vi "state buffer.vi"(8 "change command":T2, 9 "write state":T1={"command"=enum."Idle", "start time (ms)"=0, "Channel Indices"=[], "Scans per Sample"=1} {"Scans per Sample" min=1}, 10 "connection":refnum<k5>, 11 "command":T3(ring)) -> (0 "state array":T1[](array[typedef]) {"Scans per Sample" min=1}, 1 "connections":refnum<k5>[](array[refnum]), 2 "clients":i32)   [LabVIEW 2012]
uses:
  command cluster.ctl
  command.ctl
panel:
  in  "add state":T1={"command"=enum."Idle", "start time (ms)"=0, "Channel Indices"=[], "Scans per Sample"=1} {"Scans per Sample" min=1}
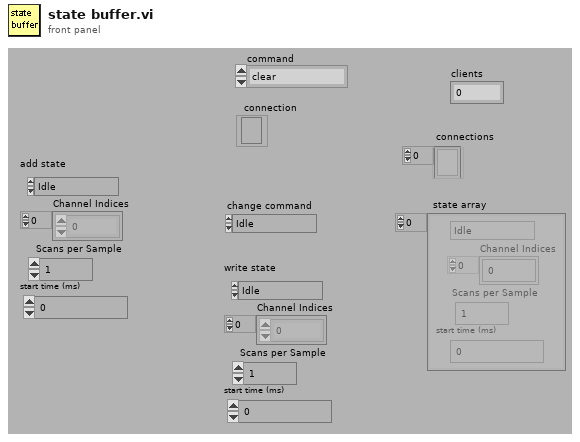
[diagram p1: front panel]
types:
  T1 = typedef "command cluster.ctl" = cluster{"command":T2, "start time (ms)":u32, "Channel Indices":i32[], "Scans per Sample":i32}
  T2 = typedef "command.ctl" = enum16{"Idle", "Send Data", "Send 1 Scan", "Logoff"}
  T3 = enum16{"clear", "add connection", "change command", "write state", "delete connection", "read"}
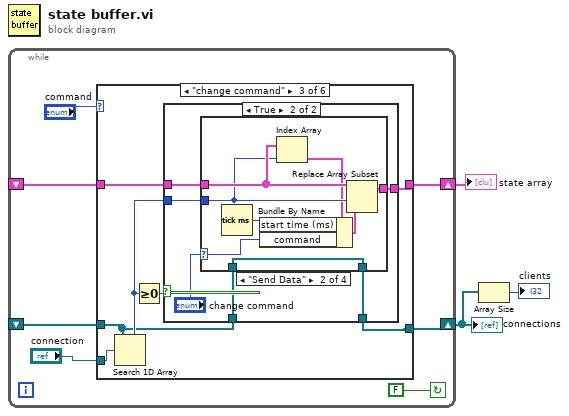
[diagram p0: block diagram]
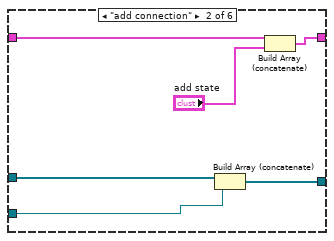
[diagram p3: hidden frame]
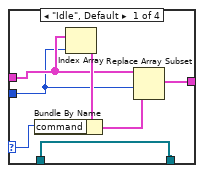
[diagram p5: hidden frame]
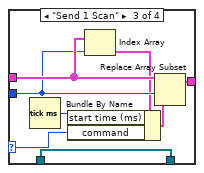
[diagram p6: hidden frame]
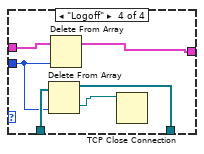
[diagram p7: hidden frame]
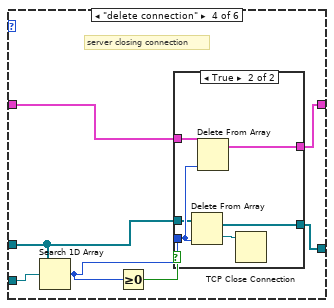
[diagram p8: hidden frame]
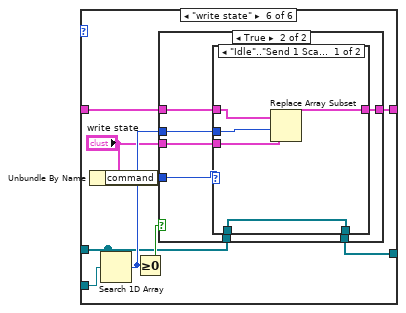
[diagram p11: hidden frame]
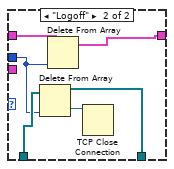
[diagram p13: hidden frame]
diagram:
  n1 = while {
    shift-right: [w10] -> w3
    shift-left: _ -> [w6]
    shift-right: [w9] -> w2
    shift-left: _ -> [w7]
    stop <- FALSE continue-if-true
    n2 = case shown="\"change command\"" "command" {
      tunnel: [_ w12 w22 w65 w77 w84] -> w10
      tunnel: [_ w15 w18 w63 w76 w80] -> w9
      tunnel: w7 -> [_ w16 w17 w64 w76 w81]
      tunnel: w6 -> [_ w13 w23 w66 w77 w85]
      tunnel: "connection" -> [_ w11 w21 w67 _ w86]
      frame "clear", Default {
      }
      frame "add connection" {
        n3 = Build Array (concatenate)(w16, w11) -> (w15:refnum<k5>[])
        n4 = Build Array (concatenate)(w13, "add state") -> (w12:T1[])
      }
      frame "change command" {
        n5 = Search 1D Array(1D array=w17, element=w21) -> (index of element=w19:i32)  [unwired: 1 in]
        n6 = Greater Or Equal To 0?(x=w19) -> (x >= 0?=w20:bool)
        n7 = case shown="True" w20 {
          tunnel: w23 -> [w25 w30]
          tunnel: w19 -> [_ w29]
          tunnel: [w25 w31] -> w22
          tunnel: w17 -> [w24 w27]
          tunnel: [w24 w26] -> w18
          frame False {
          }
          frame True {
            n8 = case shown="\"Send Data\"" "change command" {
              selector: "change command" -> [w35 w40 w48 _]
              tunnel: [w32 w46 w54 w58] -> w31
              tunnel: w30 -> [w34 w45 w53 w59]
              tunnel: w29 -> [w33 w44 w52 w56]
              tunnel: w27 -> [w38 w39 w47 w57]
              tunnel: [w38 w39 w47 w55] -> w26
              frame "Idle", Default {
                n9 = Index Array(array=w34, index=w33) -> (element=w37:T1)
                n10 = Bundle By Name(cluster=w37, "command"=w35) -> (w36:T1)
                n11 = Replace Array Subset(array=w34, new element=w36, index=w33) -> (w32:T1[])
              }
              frame "Send Data" {
                n12 = Tick Count (ms)() -> (millisecond timer value=w41:u32)
                n13 = Index Array(array=w45, index=w44) -> (element=w43:T1)
                n14 = Bundle By Name(cluster=w43, "start time (ms)"=w41, "command"=w40) -> (w42:T1)
                n15 = Replace Array Subset(array=w45, new element=w42, index=w44) -> (w46:T1[])
              }
              frame "Send 1 Scan" {
                n16 = Tick Count (ms)() -> (millisecond timer value=w49:u32)
                n17 = Index Array(array=w53, index=w52) -> (element=w51:T1)
                n18 = Bundle By Name(cluster=w51, "start time (ms)"=w49, "command"=w48) -> (w50:T1)
                n19 = Replace Array Subset(array=w53, new element=w50, index=w52) -> (w54:T1[])
              }
              frame "Logoff" {
                n20 = Delete From Array(array=w57, index=w56) -> (deleted portion=w60:refnum<k5>, array with subset deleted=w55:refnum<k5>[])  [unwired: 1 in]
                n21 = Delete From Array(array=w59, index=w56) -> (array with subset deleted=w58:T1[])  [unwired: 1 in, 1 out]
                n22 = TCP Close Connection(connection ID=w60) -> ()  [unwired: 2 in, 2 out]
              }
            }
          }
        }
      }
      frame "delete connection" {
        # "server closing connection"
        n23 = Search 1D Array(1D array=w64, element=w67) -> (index of element=w62:i32)  [unwired: 1 in]
        n24 = Greater Or Equal To 0?(x=w62) -> (x >= 0?=w61:bool)
        n25 = case shown="True" w61 {
          tunnel: w66 -> [w69 w75]
          tunnel: w62 -> [_ w74]
          tunnel: [w69 w73] -> w65
          tunnel: w64 -> [w68 w72]
          tunnel: [w68 w71] -> w63
          frame False {
          }
          frame True {
            n26 = Delete From Array(array=w72, index=w74) -> (deleted portion=w70:refnum<k5>, array with subset deleted=w71:refnum<k5>[])  [unwired: 1 in]
            n27 = Delete From Array(array=w75, index=w74) -> (array with subset deleted=w73:T1[])  [unwired: 1 in, 1 out]
            n28 = TCP Close Connection(connection ID=w70) -> ()  [unwired: 2 in, 2 out]
          }
        }
      }
      frame "read" {
      }
      frame "write state" {
        n29 = Unbundle By Name("write state") -> ("command"=w78:T2)
        n30 = Search 1D Array(1D array=w81, element=w86) -> (index of element=w82:i32)  [unwired: 1 in]
        n31 = Greater Or Equal To 0?(x=w82) -> (x >= 0?=w83:bool)
        n32 = case shown="True" w83 {
          tunnel: w85 -> [w88 w95]
          tunnel: [w88 w94] -> w84
          tunnel: "write state" -> [_ w93]
          tunnel: w82 -> [_ w92]
          tunnel: w81 -> [w87 w91]
          tunnel: [w87 w90] -> w80
          tunnel: w78 -> [_ w89]
          frame False {
          }
          frame True {
            n33 = case shown="\"Idle\"..\"Send 1 Scan\", Default" w89 {
              tunnel: w95 -> [w100 w103]
              tunnel: [w99 w101] -> w94
              tunnel: w93 -> [w98 _]
              tunnel: w92 -> [w97 w102]
              tunnel: w91 -> [w96 w105]
              tunnel: [w96 w104] -> w90
              frame "Idle".."Send 1 Scan", Default {
                n34 = Replace Array Subset(array=w100, new element=w98, index=w97) -> (w99:T1[])
              }
              frame "Logoff" {
                n35 = Delete From Array(array=w105, index=w102) -> (deleted portion=w106:refnum<k5>, array with subset deleted=w104:refnum<k5>[])  [unwired: 1 in]
                n36 = Delete From Array(array=w103, index=w102) -> (array with subset deleted=w101:T1[])  [unwired: 1 in, 1 out]
                n37 = TCP Close Connection(connection ID=w106) -> ()  [unwired: 2 in, 2 out]
              }
            }
          }
        }
      }
    }
  }
  "connections" <- w2
  "state array" <- w3
  n38 = Array Size(array=w2) -> (size(s)=→"clients":i32)
